vi "超标留样型号配置.vi"(11 "输入":T1={"确定"=FALSE, "单选按钮"=enum."德润DR803F"}) -> (3 "输出":T1={"确定"=FALSE, "单选按钮"=enum."德润DR803F"})   [LabVIEW 2016]
panel:
  in  "退出":bool
  in  "确定":bool
  in  "单选按钮":T2(radio)
  # "超标留样型号配置"
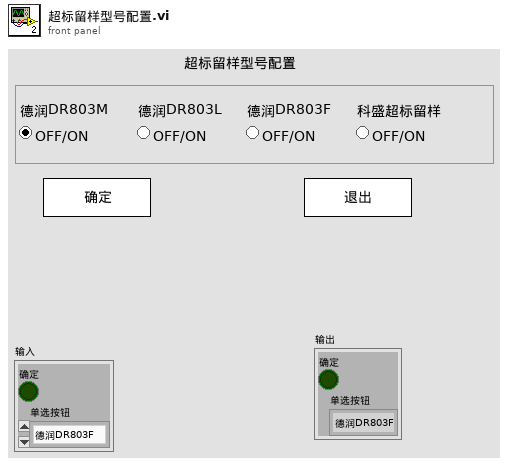
[diagram p1: front panel]
types:
  T1 = cluster{"确定":bool, "单选按钮":enum32{"德润DR803M", "德润DR803L", "德润DR803F", "科盛超标留样"}}
  T2 = enum32{"德润DR803M", "德润DR803L", "德润DR803F", "科盛超标留样"}
  T3 = cluster{"确定":bool, "单选按钮":enum32{"DR803M", "DR803L", "DR803F", "科盛超标留样"}}
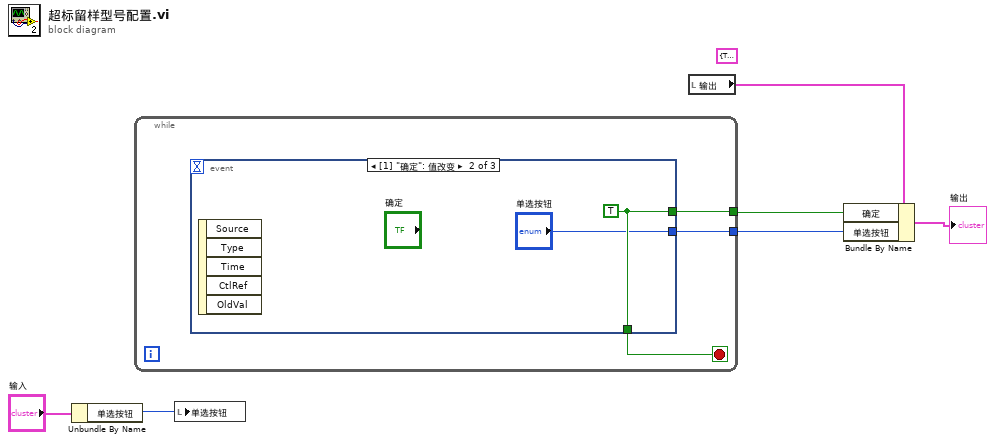
[diagram p0: block diagram]
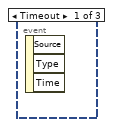
[diagram p2: hidden frame]
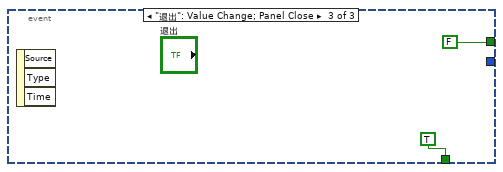
[diagram p3: hidden frame]
diagram:
  (unwired) T3 {"确定"=TRUE, "单选按钮"=enum."DR803F"}
  n1 = Unbundle By Name("输入") -> ("单选按钮"=w1:T2)
  n2 = while {
    tunnel: [w8] -> w4
    tunnel: [w7] -> w3
    stop <- w9 stop-if-true
    n3 = event shown="[1] \"确定\": 值改变" {
      selector: _ -> [_ _ _]
      dyn-events: _ -> [_ _ _]
      timeout: _ -> [_ _ _]
      tunnel: [_ w11 TRUE ("确定")] -> w9
      tunnel: [_ w11 FALSE] -> w8
      tunnel: [_ "单选按钮" _] -> w7
      event Timeout {
        n4 = event-data() -> ()  [unwired: 1 in, 3 out]
      }
      event "确定": Value Change {
        w11 = TRUE
        n5 = event-data() -> ()  [unwired: 1 in, 5 out]
      }
      event "退出": Value Change; Panel Close {
        n6 = event-data() -> ()  [unwired: 1 in, 3 out]
      }
    }
  }
  n7 = local write "单选按钮"(w1) -> ()
  n8 = local read "输出"() -> (w6:T1)
  n9 = Bundle By Name(cluster=w6, "确定"=w4, "单选按钮"=w3) -> (→"输出":T1)
